vi "Serial Read Test.vi"() -> ()   [LabVIEW 2014]
uses:
  <vilib>/Instr/_visa.llb/VISA Configure Serial Port (Instr).vi
panel:
  out "Bytes":dbl
  in  "Start":bool
  out "Read":string
  in  "VISA resource name":refnum<visa-resource-name>
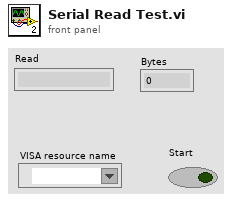
[diagram p1: front panel]
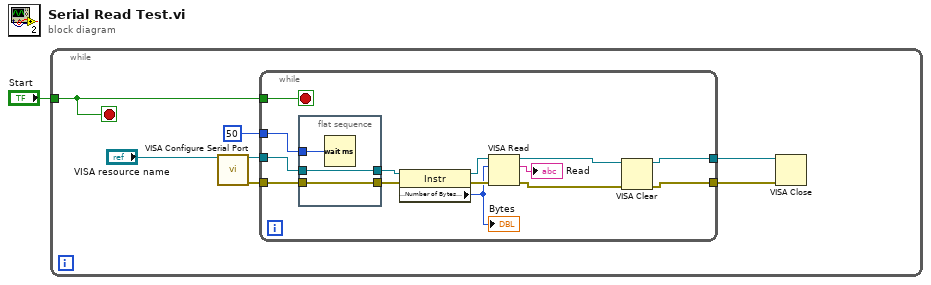
[diagram p0: block diagram]
diagram:
  n1 = while {
    tunnel: "Start" -> [w3]
    stop <- w3 stop-if-true
    n2 = call-poly "VISA Configure Serial Port"("VISA resource name"="VISA resource name") -> ("VISA resource name out"=w5:refnum<visa-resource-name>, "error out"=w4:errorcluster)  [unwired: 13 in]
    n3 = while {
      tunnel: w3 -> [w22]
      tunnel: 50 -> [w21]
      tunnel: [w11] -> w7
      tunnel: w5 -> [w20]
      tunnel: w4 -> [w14]
      tunnel: [w10] -> w2
      stop <- w22 stop-if-true
      n4 = flat-sequence {
        tunnel: w21 -> [w25]
        tunnel: w14 -> [w24]
        tunnel: [w24] -> w18
        tunnel: [w23] -> w19
        tunnel: w20 -> [w23]
        frame #0 {
          n5 = Wait (ms)(milliseconds to wait=w25) -> ()  [unwired: 1 out]
        }
      }
      n6 = property class="Instr"(reference=w19, error in=w18) -> (reference out=w16:refnum<visa-resource-name>, error out=w17:errorcluster, "Serial Settings:Number of Bytes at Serial Port"=w13:u32)
      "Bytes" <- w13
      n7 = VISA Read(VISA resource name=w16, byte count=w13, error in (no error)=w17) -> (VISA resource name out=w12:refnum<visa-resource-name>, read buffer=→"Read":string, error out=w9:errorcluster)  [unwired: 1 out]
      n8 = VISA Clear(VISA resource name=w12, error in (no error)=w9) -> (VISA resource name out=w10:refnum<visa-resource-name>, error out=w11:errorcluster)
    }
    n9 = VISA Close(VISA resource name=w2, error in (no error)=w7) -> ()  [unwired: 1 out]
  }
